vi "New.vi"(8 "error in (no error)":errorcluster, 10 "Options":string="{}", 11 "Endpoint URI":string) -> (0 "error out":errorcluster, 2 "notifier out":refnum<notifier>, 3 "Unregister JSON out":refnum<class "Unregister JSON.lvclass">)   [LabVIEW 2020, in "wamplv.lvlib" / "Unregister JSON.lvclass"]
uses:
  Unregister JSON.lvclass
  WAMP Client/Private/TypeDef/Unregister request (JSON).ctl
  Unregister JSON.lvclass/Unregister JSON.ctl
  wamplv.lvlib
  Message loop classes/ErrorOrSuccess JSON/ErrorOrSuccess JSON.lvclass
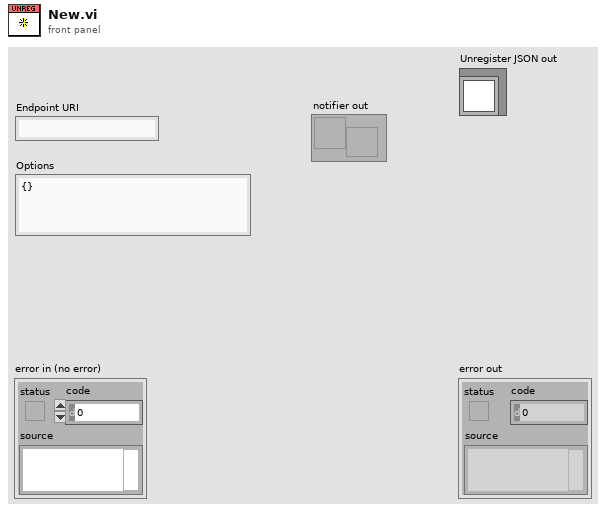
[diagram p1: front panel]
types:
  T1 = typedef "wamplv.lvlib/Unregister request (JSON).ctl" = cluster{"URI":string, "Options":string, "Unregister result notifier":refnum<notifier>}
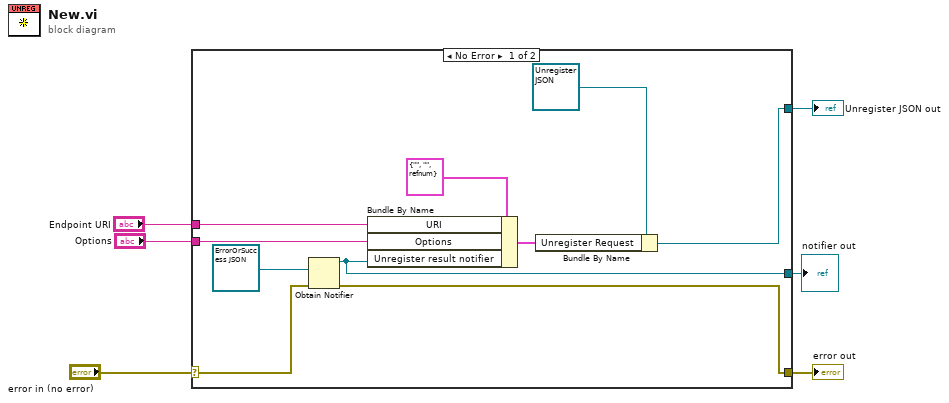
[diagram p0: block diagram]
diagram:
  n1 = case shown="No Error" "error in (no error)" {
    selector: "error in (no error)" -> [w16 w17]
    tunnel: [w9 w17] -> w5
    tunnel: [w12 _] -> w4
    tunnel: "Options" -> [w14 _]
    tunnel: "Endpoint URI" -> [w13 _]
    tunnel: [w8 _] -> w1
    frame No Error {
      n2 = Obtain Notifier(notification data type=refnum<class "ErrorOrSuccess JSON.lvclass"> refnum ("wamplv.lvlib:ErrorOrSuccess JSON.lvclass"), error in (no error)=w16) -> (notifier out=w8:refnum<notifier>, error out=w9:errorcluster)  [unwired: 2 in, 1 out]
      n3 = Bundle By Name(cluster=T1 {"URI"="", "Options"="", "Unregister result notifier"=refnum} ("Unregister Request"), "URI"=w13, "Options"=w14, "Unregister result notifier"=w8) -> (w10:T1)
      n4 = Bundle By Name(cluster=refnum<class "Unregister JSON.lvclass"> refnum ("wamplv.lvlib:Unregister JSON.lvclass"), "Unregister Request"=w10) -> (w12:refnum<class "Unregister JSON.lvclass">)
    }
    frame Error {
    }
  }
  "error out" <- w5
  "Unregister JSON out" <- w4
  "notifier out" <- w1
